vi "Signals Example.vi"() -> ()   [LabVIEW 2010]
doc: "Use this VI to measure the state, rate, level, shape, and frequency of the square wave signal generated by the DAQ Signal Accessory."
uses:
  <vilib>/express/express analysis/Spectral/XNode/ExpressSpectralMeasurementsBlockNode.xnode
  <vilib>/DAQmx/read.llb/DAQmx Read (Analog DBL 1Chan 1Samp).vi
  <vilib>/DAQmx/read.llb/DAQmx Read (Analog Wfm 1Chan NSamp).vi
  <vilib>/DAQmx/create/channels.llb/DAQmx Create Channel (AI-Voltage-Basic).vi
  <vilib>/daqmx/miscellaneous.llb/DAQmx Fill In Error Info.vi
  <vilib>/DAQmx/configure/timing.llb/DAQmx Timing (Sample Clock).vi
  <vilib>/express/express analysis/Spectral/Block/exnSpectralBlock spectral measurements power poly.vi
  <vilib>/express/express analysis/Spectral/Block/exnSpectralBlock spectral measurements power WFM.vi
panel:
  in  "stop":bool
  in  "PCI DAQ Device Channel 1":tag="cDAQ1Mod2/ai0"
  out "Time Domain":waveform(dbl)(graph)={"t0"=timestamp(3286995195.0384927 s since 1904-01-01), "dt"=0.0, "Y"=[], "attributes"=variant("NI_ChannelName"=variant(string "Analog Input 1"), "NI_UnitDescription"=variant(string "Volts"))}
  out "Frequency Domain":cluster{"f0":dbl, "df":dbl, "magnitude":dbl[]}(graph)
  out "DC Signal":dbl(graph)=-0.0003017669999999979
  in  "Signal Class":T1(ring)=enum."Analog DC"
  out "Pulse State (ON/OFF)":bool
  out "Pulses Counted":i32
  # "Instructions:\nBefore running the example, on the DAQ Signal Accessory:\n1.  Connect square wave output to Analog Input 1.\n2. Set the Frequency Range to 100Hz - 10kHz\n3. Turn the Frequency Adjust counter-clockwise until it stops.\n4. Start the VI\n5. Select the Signal Class and change the frequency adjust \nknob as desired\n6. Stop when finished"
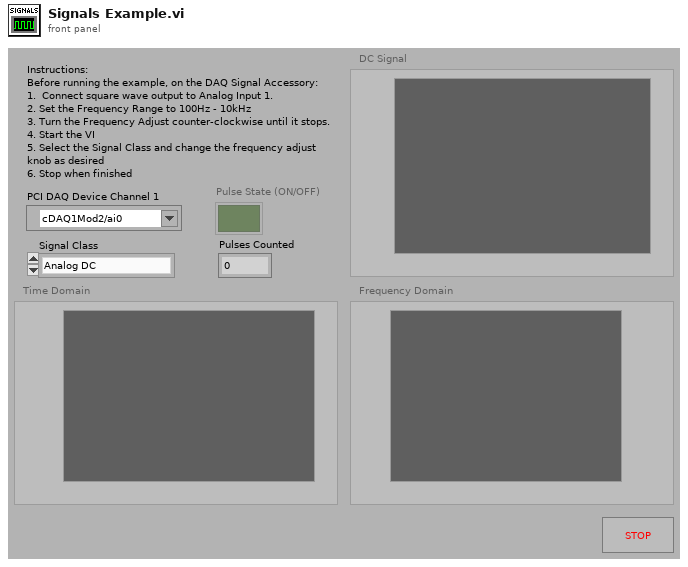
[diagram p1: front panel]
types:
  T1 = enum16{"Digital On/Off", "Digital Pulse Train", "Analog DC", "Time Domain", "Frequency Domain"}
  T2 = cluster{"averaging mode":u16, "weighting mode":u16, "number of averages":u32}
  T3 = cluster{"dB On (F)":bool, "unwrap phase (F)":bool, "convert to degree (F)":bool}
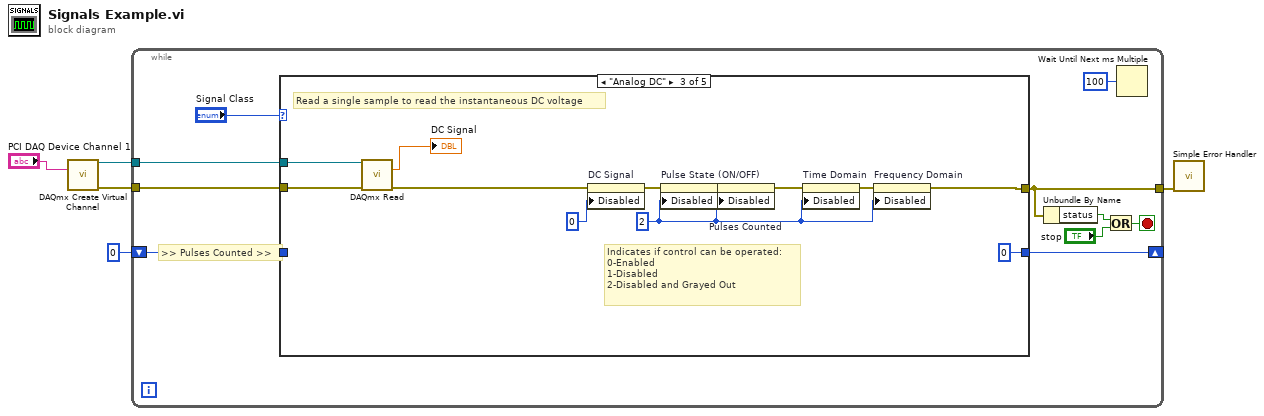
[diagram p0: block diagram]
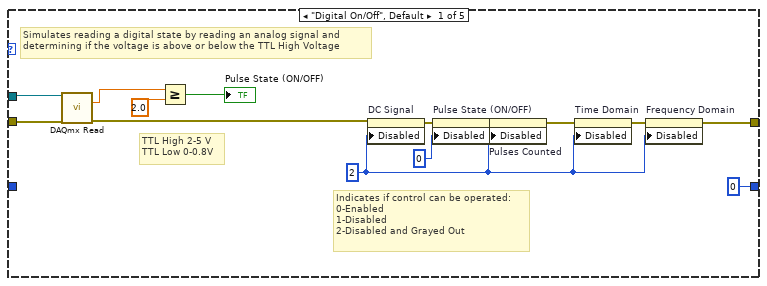
[diagram p2: hidden frame]
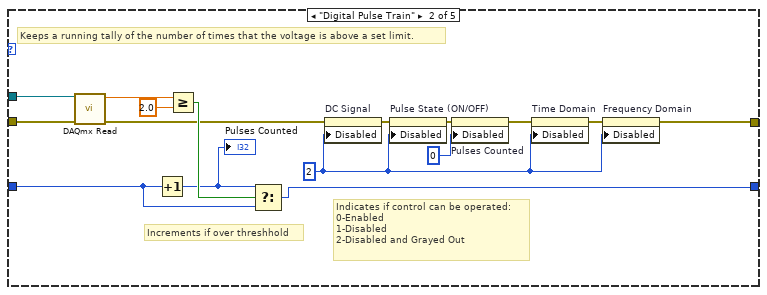
[diagram p3: hidden frame]
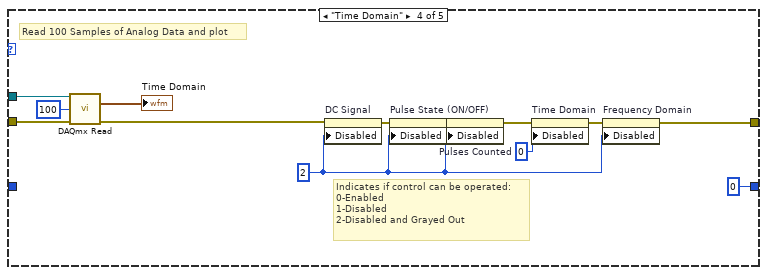
[diagram p4: hidden frame]
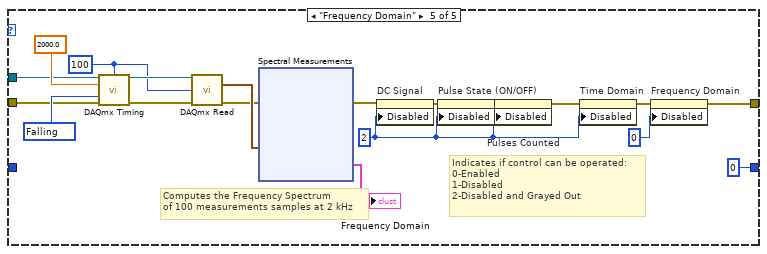
[diagram p5: hidden frame]
diagram:
  n1 = call-poly <vilib>:"DAQmx Create Virtual Channel.vi"("physical channels"="PCI DAQ Device Channel 1") -> ("task out"=w4:refnum<k21>, "error out"=w3:errorcluster)  [unwired: 13 in]
  n2 = while {
    tunnel: w4 -> [w15]
    tunnel: w3 -> [w14]
    tunnel: [w11] -> w1
    shift-right: [w10] -> _
    shift-left: 0 -> [w13]
    stop <- w8 stop-if-true
    # ">> Pulses Counted >>"
    n3 = case shown="\"Analog DC\"" "Signal Class" {
      tunnel: [w24 w31 w49 w66 w85] -> w11
      tunnel: w15 -> [w19 w41 w48 w62 w78]
      tunnel: w14 -> [w20 w40 w47 w63 w77]
      tunnel: w13 -> [_ w39 _ _ _]
      tunnel: [0 w38 0 0 0] -> w10
      frame "Digital On/Off", Default {
        w29 = u8 2 ("Disabled")
        # "Indicates if control can be operated: \n0-Enabled\n1-Disabled \n2-Disabled and Grayed Out"
        # "Simulates reading a digital state by reading an analog signal and \ndetermining if the voltage is above or below the TTL High Voltage"
        # "TTL High 2-5 V\nTTL Low 0-0.8V"
        n4 = call-poly <vilib>:"DAQmx Read.vi"("task/channels in"=w19, "error in"=w20) -> ("data"=w21:dbl, "error out"=w18:errorcluster)  [unwired: 11 in, 1 out]
        n5 = Greater Or Equal?(x=w21, y=2.0) -> (x >= y?=→"Pulse State (ON/OFF)":bool)
        n6 = property on="DC Signal" class="GraphDér (strict)"(error in=w18, "Disabled"=w29) -> (error out=w25:errorcluster)  [unwired: 1 in, 1 out]
        n7 = property on="Pulse State (ON/OFF)" class="Bool (strict)"(error in=w25, "Disabled"=u8 0) -> (error out=w26:errorcluster)  [unwired: 1 in, 1 out]
        n8 = property on="Pulses Counted" class="NumDig (strict)"(error in=w26, "Disabled"=w29) -> (error out=w27:errorcluster)  [unwired: 1 in, 1 out]
        n9 = property on="Time Domain" class="GraphWF (strict)"(error in=w27, "Disabled"=w29) -> (error out=w28:errorcluster)  [unwired: 1 in, 1 out]
        n10 = property on="Frequency Domain" class="GraphWF (strict)"(error in=w28, "Disabled"=w29) -> (error out=w24:errorcluster)  [unwired: 1 in, 1 out]
      }
      frame "Digital Pulse Train" {
        w37 = u8 2 ("Disabled")
        # "Indicates if control can be operated: \n0-Enabled\n1-Disabled \n2-Disabled and Grayed Out"
        # "Keeps a running tally of the number of times that the voltage is above a set limit."
        # "Increments if over threshhold"
        n11 = call-poly <vilib>:"DAQmx Read.vi"("task/channels in"=w41, "error in"=w40) -> ("data"=w42:dbl, "error out"=w36:errorcluster)  [unwired: 11 in, 1 out]
        n12 = Increment(x=w39) -> (x+1=w44:i32)
        "Pulses Counted" <- w44
        n13 = Greater Or Equal?(x=w42, y=2.0) -> (x >= y?=w45:bool)
        n14 = Select(t=w44, s=w45, f=w39) -> (s? t:f=w38:i32)
        n15 = property on="DC Signal" class="GraphDér (strict)"(error in=w36, "Disabled"=w37) -> (error out=w35:errorcluster)  [unwired: 1 in, 1 out]
        n16 = property on="Pulse State (ON/OFF)" class="Bool (strict)"(error in=w35, "Disabled"=w37) -> (error out=w34:errorcluster)  [unwired: 1 in, 1 out]
        n17 = property on="Pulses Counted" class="NumDig (strict)"(error in=w34, "Disabled"=u8 0) -> (error out=w33:errorcluster)  [unwired: 1 in, 1 out]
        n18 = property on="Time Domain" class="GraphWF (strict)"(error in=w33, "Disabled"=w37) -> (error out=w32:errorcluster)  [unwired: 1 in, 1 out]
        n19 = property on="Frequency Domain" class="GraphWF (strict)"(error in=w32, "Disabled"=w37) -> (error out=w31:errorcluster)  [unwired: 1 in, 1 out]
      }
      frame "Analog DC" {
        w51 = u8 2 ("Disabled")
        # "Indicates if control can be operated: \n0-Enabled\n1-Disabled \n2-Disabled and Grayed Out"
        # "Read a single sample to read the instantaneous DC voltage"
        n20 = call-poly <vilib>:"DAQmx Read.vi"("task/channels in"=w48, "error in"=w47) -> ("data"=→"DC Signal":dbl, "error out"=w57:errorcluster)  [unwired: 11 in, 1 out]
        n21 = property on="DC Signal" class="GraphDér (strict)"(error in=w57, "Disabled"=u8 0) -> (error out=w53:errorcluster)  [unwired: 1 in, 1 out]
        n22 = property on="Pulse State (ON/OFF)" class="Bool (strict)"(error in=w53, "Disabled"=w51) -> (error out=w54:errorcluster)  [unwired: 1 in, 1 out]
        n23 = property on="Pulses Counted" class="NumDig (strict)"(error in=w54, "Disabled"=w51) -> (error out=w55:errorcluster)  [unwired: 1 in, 1 out]
        n24 = property on="Time Domain" class="GraphWF (strict)"(error in=w55, "Disabled"=w51) -> (error out=w56:errorcluster)  [unwired: 1 in, 1 out]
        n25 = property on="Frequency Domain" class="GraphWF (strict)"(error in=w56, "Disabled"=w51) -> (error out=w49:errorcluster)  [unwired: 1 in, 1 out]
      }
      frame "Time Domain" {
        w59 = u8 2 ("Disabled")
        # "Read 100 Samples of Analog Data and plot"
        # "Indicates if control can be operated: \n0-Enabled\n1-Disabled \n2-Disabled and Grayed Out"
        n26 = call-poly <vilib>:"DAQmx Read.vi"("task/channels in"=w62, "number of samples per channel"=100, "error in"=w63) -> ("data"=→"Time Domain":waveform(dbl), "error out"=w61:errorcluster)  [unwired: 10 in, 1 out]
        n27 = property on="DC Signal" class="GraphDér (strict)"(error in=w61, "Disabled"=w59) -> (error out=w67:errorcluster)  [unwired: 1 in, 1 out]
        n28 = property on="Pulse State (ON/OFF)" class="Bool (strict)"(error in=w67, "Disabled"=w59) -> (error out=w68:errorcluster)  [unwired: 1 in, 1 out]
        n29 = property on="Pulses Counted" class="NumDig (strict)"(error in=w68, "Disabled"=w59) -> (error out=w69:errorcluster)  [unwired: 1 in, 1 out]
        n30 = property on="Time Domain" class="GraphWF (strict)"(error in=w69, "Disabled"=u8 0) -> (error out=w70:errorcluster)  [unwired: 1 in, 1 out]
        n31 = property on="Frequency Domain" class="GraphWF (strict)"(error in=w70, "Disabled"=w59) -> (error out=w66:errorcluster)  [unwired: 1 in, 1 out]
      }
      frame "Frequency Domain" {
        w83 = u8 2 ("Disabled")
        w81 = 10171 items=["Rising"=10280, "Falling"=10171] ("active edge")
        w76 = 100 ("samples per channel")
        # "Computes the Frequency Spectrum \nof 100 measurements samples at 2 kHz"
        # "Indicates if control can be operated: \n0-Enabled\n1-Disabled \n2-Disabled and Grayed Out"
        n32 = call-poly <vilib>:"DAQmx Timing.vi"("task/channels in"=w78, "samples per channel"=w76, "rate"=2000.0, "active edge"=w81, "error in"=w77) -> ("task out"=w79:refnum<k21>, "error out"=w80:errorcluster)  [unwired: 9 in]
        n33 = call-poly <vilib>:"DAQmx Read.vi"("task/channels in"=w79, "number of samples per channel"=w76, "error in"=w80) -> ("data"=w75:waveform(dbl), "error out"=w73:errorcluster)  [unwired: 10 in, 1 out]
        n34 = xnode "Spectral Measurements"("Signaux"=w75, "entrée d'erreur (pas d'erreur)"=w73) -> ("Power Spectrum"=→"Frequency Domain":cluster{"f0":dbl, "df":dbl, "magnitude":dbl[]}, "sortie d'erreur"=w72:errorcluster)
        n35 = property on="DC Signal" class="GraphDér (strict)"(error in=w72, "Disabled"=w83) -> (error out=w86:errorcluster)  [unwired: 1 in, 1 out]
        n36 = property on="Pulse State (ON/OFF)" class="Bool (strict)"(error in=w86, "Disabled"=w83) -> (error out=w87:errorcluster)  [unwired: 1 in, 1 out]
        n37 = property on="Pulses Counted" class="NumDig (strict)"(error in=w87, "Disabled"=w83) -> (error out=w88:errorcluster)  [unwired: 1 in, 1 out]
        n38 = property on="Time Domain" class="GraphWF (strict)"(error in=w88, "Disabled"=w83) -> (error out=w89:errorcluster)  [unwired: 1 in, 1 out]
        n39 = property on="Frequency Domain" class="GraphWF (strict)"(error in=w89, "Disabled"=u8 0) -> (error out=w85:errorcluster)  [unwired: 1 in, 1 out]
      }
    }
    n40 = Unbundle By Name(w11) -> ("status"=w9:bool)
    n41 = Or(x=w9, y="stop") -> (x .or. y?=w8:bool)
    n42 = Wait Until Next ms Multiple(millisecond multiple=u32 100) -> ()  [unwired: 1 out]
  }
  n43 = call <vilib>:"Simple Error Handler.vi"("error in (no error)"=w1) -> ()  [unwired: 4 in, 5 out]
